vi "JamesBroad.vi"(8 "error in (no error)":errorcluster, 9 "String":string, 11 "TemplateModule in":refnum<class "TemplateModule.lvclass">) -> (0 "error out":errorcluster, 3 "TemplateModule out":refnum<class "TemplateModule.lvclass">)   [LabVIEW 2024, in "TemplateModule.lvclass"]
uses:
  TemplateModule.lvclass
  JamesBroad.ctl
  RQMHCore/ModuleCore/RQMHModule.lvclass
  TemplateModule.lvclass/TemplateModule.ctl
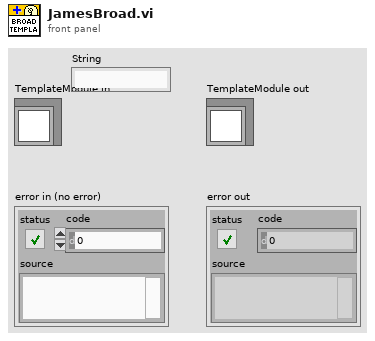
[diagram p1: front panel]
types:
  T1 = typedef "TemplateModule.lvclass/JamesBroad.ctl" = cluster{"Module":refnum<class "RQMHModule.lvclass">, "String":string}
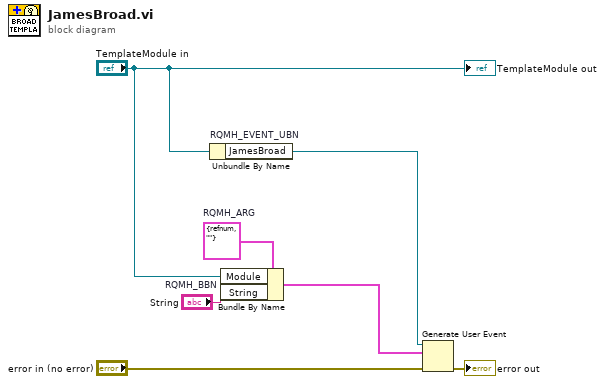
[diagram p0: block diagram]
diagram:
  w4 = T1 {"Module"=refnum, "String"=""}  # RQMH_ARG
  n1 = Unbundle By Name "RQMH_EVENT_UBN"("TemplateModule in") -> ("JamesBroad"=w7:refnum<user-event>)
  n2 = Bundle By Name "RQMH_BBN"(cluster=w4, "Module"="TemplateModule in", "String"="String") -> (w3:T1)
  n3 = Generate User Event(user event=w7, event data cluster=w3, error in="error in (no error)") -> (error out=→"error out":errorcluster)  [unwired: 1 in, 1 out]
  "TemplateModule out" <- "TemplateModule in"
